vi "YTO_CLR_unlock_Naoj.vi"(5 "Cartridge band":u32 max=10 step=1, 7 "Slave Node in":cluster{"Address":i16, "Serial Number":i8[]}={"Address"=19, "Serial Number"=[16, 71, 55, 76, 1, 8, 0, -15]} {"Serial Number" format="%.0x"; "Address" format="%.0x"}, 8 "error IO":errorcluster, 11 "ObjHandle in":u32) -> (0 "error":errorcluster, 3 "ObjHandle out":u32)   [LabVIEW 2017]
panel:
  # "Node Address"
  # "Serial Number"
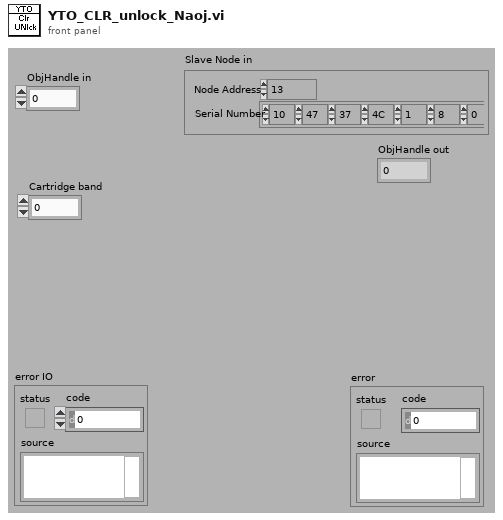
[diagram p1: front panel]
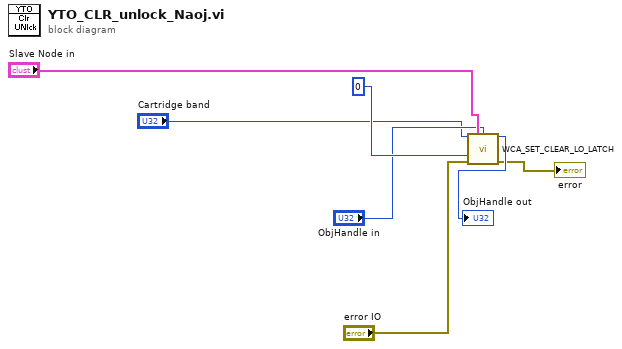
[diagram p0: block diagram]
diagram:
  n1 = call "WCA_SET_CLEAR_LO_LATCH.vi"("Cartridge Band"="Cartridge band", "Slave Node in"="Slave Node in", "ObjHandle in"="ObjHandle in", "SET_CLEAR_LO_LATCH"=0 ("SET CLEAR LO LATCH"), "error in (no error)"="error IO") -> ("ObjHandle out"=→"ObjHandle out":u32, "error out"=→"error":errorcluster)  [unwired: 9 in]
